vi "Stable.vi"(1 "last 20 field numbers":dbl[unit][](array[numeric])) -> (0 "Stable?":bool)   [LabVIEW 2009, in "Varian.lvlib"]
uses:
  Varian.lvlib
  <vilib>/Analysis/NI_AALBase.lvlib
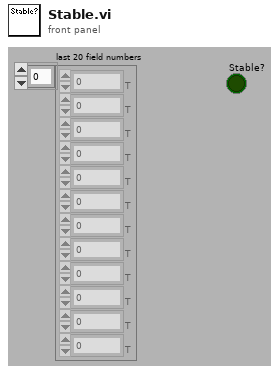
[diagram p1: front panel]
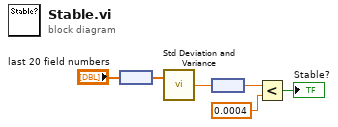
[diagram p0: block diagram]
diagram:
  n1 = node("last 20 field numbers") -> (w3:dbl[])
  n2 = call <vilib>:"Std Deviation and Variance.vi"("X"=w3) -> ("standard deviation"=w6:dbl)  [unwired: 1 in, 2 out]
  n3 = node(w6) -> (w2:dbl[unit])
  n4 = Less?(x=w2, y=dbl[unit] 0.0004 ("x")) -> (x < y?=→"Stable?":bool)
